vi "test Pointer Lifecycle.vi"(8 "error in (no error)":errorcluster, 11 "Test Case in":refnum<class "Lifecycle Tests.lvclass">) -> (0 "error out":errorcluster, 3 "Test Case out":refnum<class "Lifecycle Tests.lvclass">)   [LabVIEW 2017, in "Pointer Tests.lvlib" / "Lifecycle Tests.lvclass"]
uses:
  Lifecycle Tests/Lifecycle Tests.lvclass
  Source/Classes/Pointer/Pointer.lvclass
  Source/Classes/Pointer/Public/New/New (1B).vi
  <vilib>/addons/_JKI Toolkits/VI Tester/TestCase.llb/TestCase.lvclass
  C:/Program Files (x86)/National Instruments/LabVIEW 2017/vi.lib/addons/_JKI Toolkits/VI Tester/TestCase.llb/TestCase.lvclass
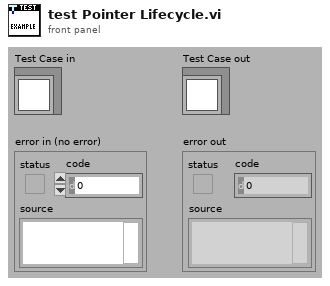
[diagram p1: front panel]
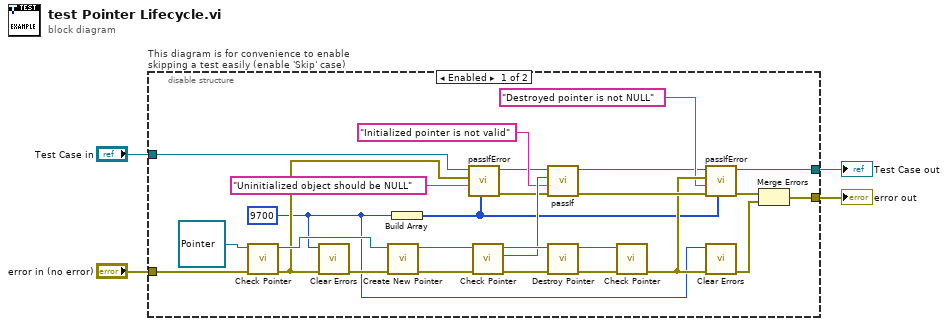
[diagram p0: block diagram]
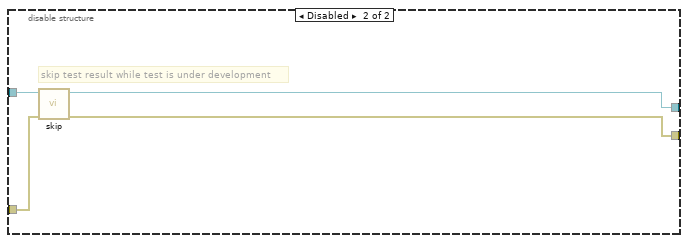
[diagram p2: hidden frame]
diagram:
  n1 = disable-structure "This diagram is for convenience to enable skipping a test easily (enable 'Skip' case)" shown="Enabled" {
    disable-tunnel: "Test Case in" -> [w11 w35]
    disable-tunnel: [w12 w33] -> w2
    disable-tunnel: [w21 w34] -> w1
    disable-tunnel: "error in (no error)" -> [w7 w32]
    frame Enabled {
      w8 = 9700 ("pass error code (0=any error code)")
      n2 = call "Check Pointer.vi"("error in (no error)"=w7, "Pointer in"=refnum<class "Pointer.lvclass"> refnum) -> ("error out"=w17:errorcluster, "Pointer out"=w29:refnum<class "Pointer.lvclass">)  [unwired: 7 in, 1 out]
      n3 = call <vilib>:"Clear Errors.vi"("error in (no error)"=w17, "specific error code to clear (0: all)"=w8) -> ("error out"=w16:errorcluster)  [unwired: 4 in, 1 out]
      n4 = call-poly "Create New Pointer.vi"("error in (no error)"=w16, "Pointer type"=w29) -> ("error out"=w27:errorcluster, "Pointer"=w28:refnum<class "Pointer.lvclass">)  [unwired: 8 in]
      n5 = Build Array(w8) -> (w9:i32[])
      n6 = call-dynamic "passIfError.vi"("passing error codes (default = any error code)"=w9, "task (\"\")"="Uninitialized object should be NULL" ("task (\"\")"), "error"=w17, "TestCase in"=w11) -> ("error out"=w24:errorcluster, "TestCase out"=w10:refnum<class "Lifecycle Tests.lvclass">)  [unwired: 6 in]
      n7 = call "Check Pointer.vi"("error in (no error)"=w27, "Pointer in"=w28) -> ("error out"=w5:errorcluster, "LabVIEW pointer?"=w25:bool, "Pointer out"=w26:refnum<class "Pointer.lvclass">)  [unwired: 7 in]
      n8 = call-dynamic "passIf.vi"("error in (no error)"=w24, "message (\"\")"="Initialized pointer is not valid" ("task (\"\")"), "pass"=w25, "TestCase in"=w10) -> ("error out"=w23:errorcluster, "TestCase out"=w13:refnum<class "Lifecycle Tests.lvclass">)  [unwired: 6 in]
      n9 = call "Destroy Pointer.vi"("error in (no error)"=w5, "Pointer in"=w26) -> ("error out"=w18:errorcluster, "Pointer out"=w19:refnum<class "Pointer.lvclass">)  [unwired: 8 in]
      n10 = call "Check Pointer.vi"("error in (no error)"=w18, "Pointer in"=w19) -> ("error out"=w20:errorcluster)  [unwired: 7 in, 2 out]
      n11 = call-dynamic "passIfError.vi"("passing error codes (default = any error code)"=w9, "error in (no error)"=w23, "task (\"\")"="Destroyed pointer is not NULL" ("task (\"\")"), "error"=w20, "TestCase in"=w13) -> ("error out"=w22:errorcluster, "TestCase out"=w12:refnum<class "Lifecycle Tests.lvclass">)  [unwired: 5 in]
      n12 = call <vilib>:"Clear Errors.vi"("error in (no error)"=w20, "specific error code to clear (0: all)"=w8) -> ("error out"=w6:errorcluster)  [unwired: 4 in, 1 out]
      n13 = Merge Errors(w22, w6) -> (w21:errorcluster)
    }
    frame Disabled {
      # "skip test result while test is under development"
      n14 = call <vilib>:"skip.vi"("error in (no error)"=w32, "TestCase in"=w35) -> ("error out"=w34:errorcluster, "TestCase out"=w33:refnum<class "Lifecycle Tests.lvclass">)  [unwired: 8 in]
    }
  }
  "error out" <- w1
  "Test Case out" <- w2
